vi "Query Network Hostname.vi"(8 "error in (no error)":errorcluster, 11 "VISA resource name":refnum<visa-resource-name>) -> (0 "error out":errorcluster, 2 "Network Hostname":string, 3 "VISA resource name out":refnum<visa-resource-name>)   [LabVIEW 2015, in "Rohde&Schwarz CMXP Base.lvlib"]
doc: "Queries the host name (computer name) of the R&S CMX500. The host name is part of the VISA address string for LAN-based connections.\n\nAttribute:\nRSCMXPBASE_ATTR_QUERY_NETWORK_HOSTNAME\n\nRemote-control command:\nSYSTem:COMMunicate:NET:HOSTname?"
uses:
  <instrlib>/Rohde&Schwarz CMXP Base/Rohde&Schwarz CMXP Base.lvlib
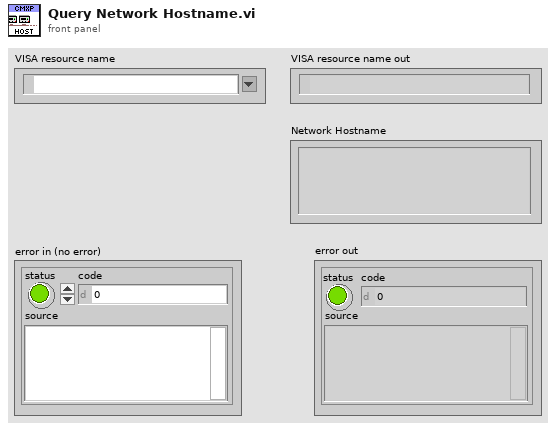
[diagram p1: front panel]
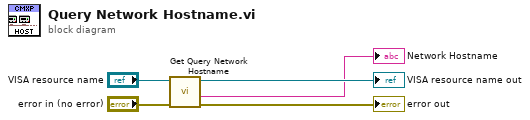
[diagram p0: block diagram]
diagram:
  n1 = call "Get Query Network Hostname"("error in (no error)"="error in (no error)", "instrument handle"="VISA resource name") -> ("error out"=→"error out":errorcluster, "Query Network Hostname"=→"Network Hostname":string, "instrument handle out"=→"VISA resource name out":refnum<visa-resource-name>)  [unwired: 7 in]
